vi "DeQueue.vi"(7 "QueName":string="BaseVisQue", 8 "Error":errorcluster[](array[cluster])) -> (0 "Error":errorcluster[](array[cluster]), 1 "Data":variant, 2 "Message":string)   [LabVIEW 2014, in "Visualization.lvlib" / "VisualizeBase_class.lvclass"]
uses:
  VisializeBase_class/VisualizeBase_class.lvclass
  Typedefs/MsgType.ctl
  <userlib>/NIST/NISTErrorLib/NISTErrorLib.lvlib
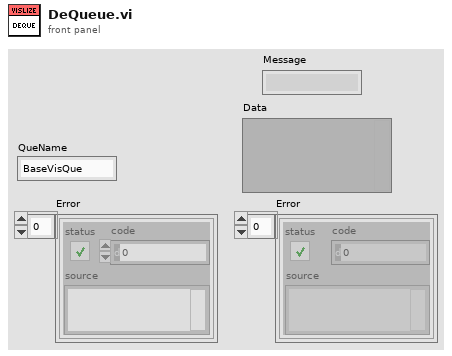
[diagram p1: front panel]
types:
  T1 = typedef "Visualization.lvlib/VisualizeBase_class.lvclass/MsgType.ctl" = cluster{"Message":string, "Data":variant}
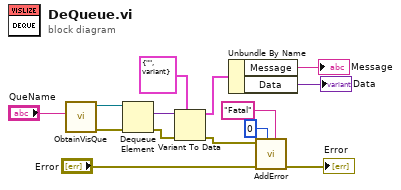
[diagram p0: block diagram]
diagram:
  n1 = call "ObtainVisQue.vi"("QueName"="QueName") -> ("error out"=w13:errorcluster, "queue out"=w14:refnum<queue>)  [unwired: 9 in]
  n2 = Dequeue Element(queue=w14, error in (no error)=w13) -> (element=w12:variant, error out=w11:errorcluster)  [unwired: 1 in, 2 out]
  n3 = Variant To Data(error in=w11, type=T1 {"Message"="", "Data"=variant} ("clMsgType"), Variant=w12) -> (data=w9:T1, error out=w6:errorcluster)
  n4 = Unbundle By Name(w9) -> ("Message"=→"Message":string, "Data"=→"Data":variant)
  n5 = call <userlib>:"AddError.vi"("Severity"="Fatal" ("String"), "Priority"=u8 0, "ErrorArray"="Error", "error in (no error)"=w6) -> ("ErrorArray"=→"Error":errorcluster[])  [unwired: 6 in, 1 out]
